vi "Stability Checker.vi"(6 "Estabilization Time":dbl, 8 "Valid Range":dbl, 9 "Setpoint":dbl, 10 "Process Variable":dbl, 11 "Start Time In":dbl) -> (1 "Is Stable":bool, 3 "Start Time Out":dbl)   [LabVIEW 2020]
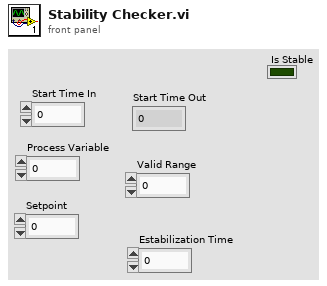
[diagram p1: front panel]
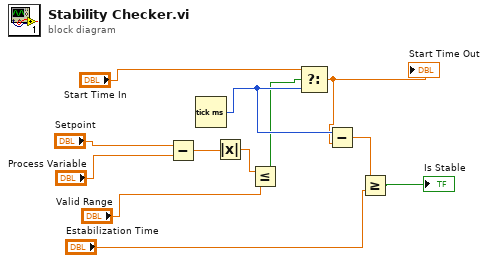
[diagram p0: block diagram]
diagram:
  n1 = Subtract(x="Setpoint", y="Process Variable") -> (x-y=w10:dbl)
  n2 = Tick Count (ms)() -> (millisecond timer value=w12:u32)
  n3 = Absolute Value(x=w10) -> (abs(x)=w9:dbl)
  n4 = Less Or Equal?(x=w9, y="Valid Range") -> (x <= y?=w7:bool)
  n5 = Select(t="Start Time In", s=w7, f=w12) -> (s? t:f=w2:dbl)
  "Start Time Out" <- w2
  n6 = Subtract(x=w12, y=w2) -> (x-y=w11:dbl)
  n7 = Greater Or Equal?(x=w11, y="Estabilization Time") -> (x >= y?=→"Is Stable":bool)
